vi "Reference - Copy and Paste Buffer.vi"(9 "Cluster2":T1, 10 "Enum":enum16{"Initialize", "Copy", "Paste"}(ring), 11 "DB Refnums":T2) -> (0 "error out":errorcluster)   [LabVIEW 2013]
uses:
  Controls/DB - Refnums.ctl
  Controls/Setup - Part Details - Item Details.ctl
  Controls/Combo Box.ctl
panel:
  out "Array 2":bool[](array[boolean])
  out "Array":bool[](array[boolean])
  out "size(s) 2":i32
  out "size(s)":i32
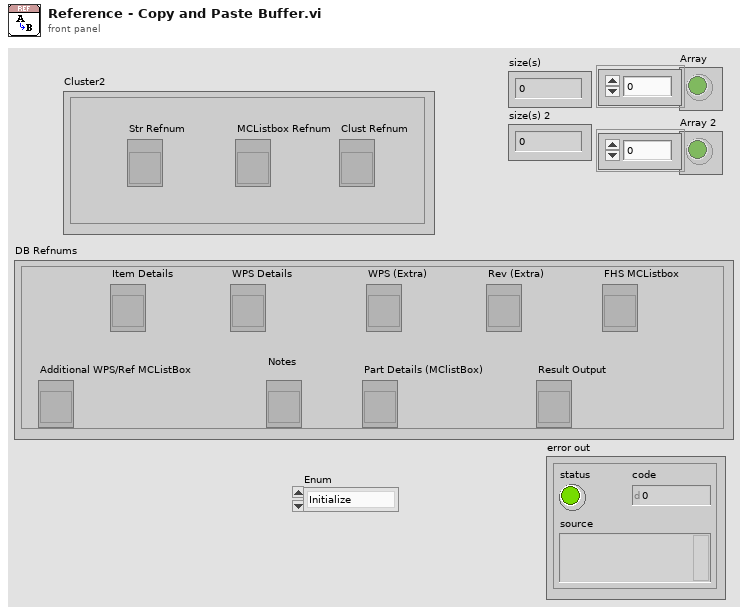
[diagram p1: front panel]
types:
  T1 = cluster{"Str Refnum":refnum<vi>, "MCListbox Refnum":refnum<vi>, "Clust Refnum":refnum<vi>}
  T2 = typedef "DB - Refnums.ctl" = cluster{"Item Details":refnum<vi>, "WPS Details":refnum<vi>, "WPS (Extra)":refnum<vi>, "Rev (Extra) ":refnum<vi>, "FHS MCListbox":refnum<vi>, "Additional WPS/Ref MCListBox":refnum<vi>, "Notes":refnum<vi>, "Part Details (MClistBox)":refnum<vi>, "Result Output":refnum<vi>}
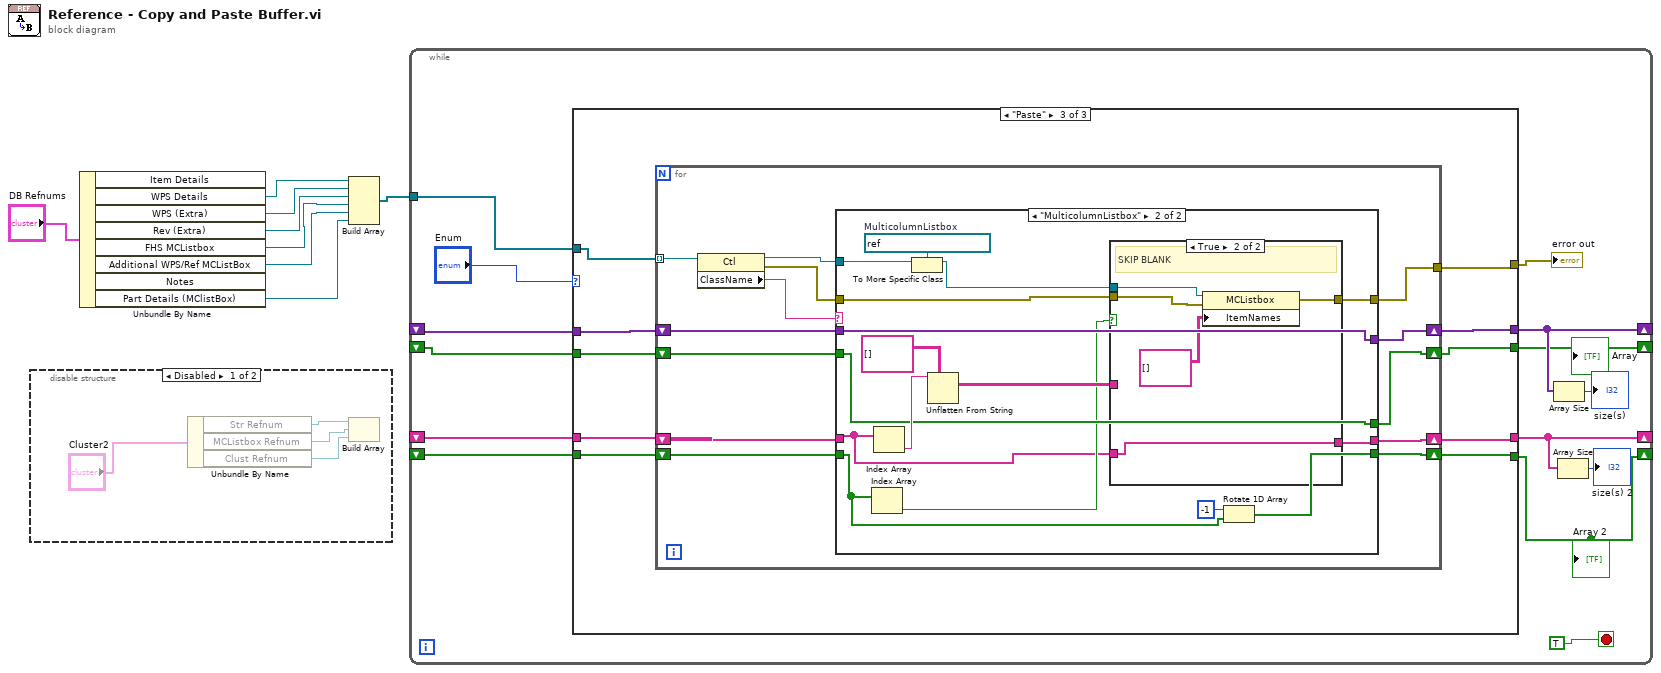
[diagram p0: block diagram]
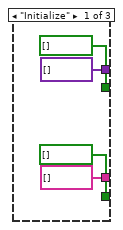
[diagram p3: hidden frame]
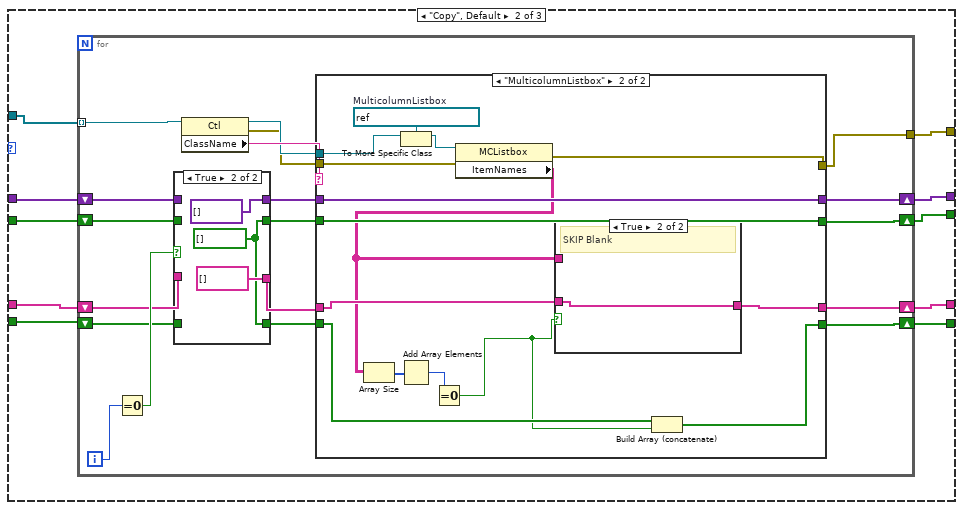
[diagram p4: hidden frame]
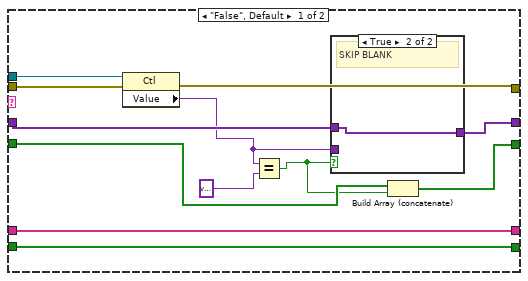
[diagram p6: hidden frame]
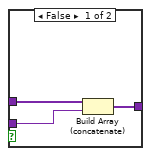
[diagram p7: hidden frame]
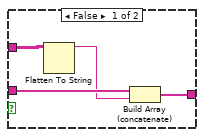
[diagram p8: hidden frame]
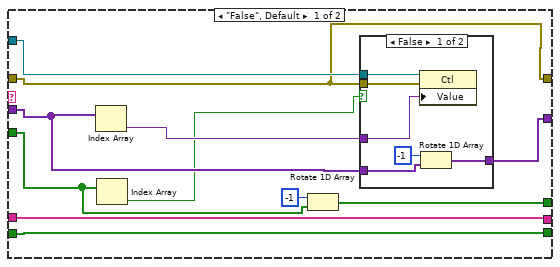
[diagram p9: hidden frame]
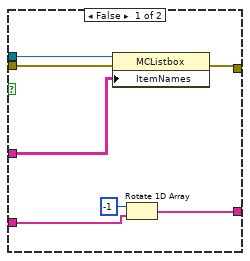
[diagram p11: hidden frame]
diagram:
  n1 = disable-structure shown="Disabled" {
    frame Disabled {
      n2 = Unbundle By Name("Cluster2") -> ("Str Refnum"=w11:refnum<vi>, "MCListbox Refnum"=w10:refnum<vi>, "Clust Refnum"=w9:refnum<vi>)
      n3 = Build Array(w11, w10, w9) -> ()  [unwired: 1 out]
    }
    frame Enabled {
    }
  }
  n4 = Unbundle By Name("DB Refnums") -> ("WPS Details"=w7:refnum<vi>, "WPS (Extra)"=w6:refnum<vi>, "Rev (Extra)"=w5:refnum<vi>, "FHS MCListbox"=w4:refnum<vi>, "Additional WPS/Ref MCListBox"=w3:refnum<vi>, "Part Details (MClistBox)"=w2:refnum<vi>)  [unwired: 2 out]
  n5 = Build Array(w7, w6, w5, w4, w3, w2) -> (w1:refnum<vi>[])
  n6 = while {
    tunnel: w1 -> [w24]
    shift-right: [w20] -> _
    shift-left: _ -> [w23]
    shift-right: [w18] -> _
    shift-left: _ -> [w22]
    shift-right: [w15] -> _
    shift-left: _ -> [w16]
    shift-right: [w13] -> _
    shift-left: _ -> [w14]
    stop <- TRUE stop-if-true
    n7 = case shown="\"Paste\"" "Enum" {
      tunnel: w24 -> [_ w35 w112]
      tunnel: [variant[] [] w40 w109] -> w20
      tunnel: w23 -> [_ w38 w111]
      tunnel: [string[] [] w39 w107] -> w18
      tunnel: w22 -> [_ w37 w108]
      tunnel: [_ w36 w110] -> w21
      tunnel: w16 -> [_ w34 w106]
      tunnel: [bool[] [] w33 w103] -> w15
      tunnel: w14 -> [_ w32 w105]
      tunnel: [bool[] [] w31 w104] -> w13
      frame "Initialize" {
      }
      frame "Copy", Default {
        n8 = for {
          tunnel: w35 -> [w59] mode=indexing
          tunnel: [w53] -> w36
          shift-right: [w54] -> w40
          shift-left: w38 -> [w51]
          shift-right: [w56] -> w39
          shift-left: w37 -> [w49]
          shift-right: [w44] -> w33
          shift-left: w34 -> [w46]
          shift-right: [w41] -> w31
          shift-left: w32 -> [w43]
          i -> [w52]
          n9 = Equal To 0?(x=w52) -> (x = 0?=w50:bool)
          n10 = case shown="True" w50 {
            tunnel: w51 -> [w63 _]
            tunnel: w49 -> [w62 _]
            tunnel: [w63 variant[] []] -> w48
            tunnel: [w62 string[] []] -> w47
            tunnel: w46 -> [w61 _]
            tunnel: [w61 w64] -> w45
            tunnel: w43 -> [w60 _]
            tunnel: [w60 w64] -> w42
            frame False {
            }
            frame True {
              w64 = bool[] []
            }
          }
          n11 = property class="Ctl"(reference=w59) -> (reference out=w57:refnum<vi>, error out=w55:errorcluster, "ClassName"=w58:string)  [unwired: 1 in]
          n12 = case shown="\"MulticolumnListbox\"" w58 {
            tunnel: w57 -> [w78 w97]
            tunnel: [w73 w91] -> w56
            tunnel: w55 -> [w77 w94]
            tunnel: [w76 w93] -> w53
            tunnel: [w74 w90] -> w54
            tunnel: w48 -> [w75 w90]
            tunnel: w47 -> [w73 w92]
            tunnel: w45 -> [w70 w87]
            tunnel: [w68 w87] -> w44
            tunnel: w42 -> [w67 w85]
            tunnel: [w67 w83] -> w41
            frame "False", Default {
              n13 = property class="Ctl"(reference=w78, error in=w77) -> (error out=w76:errorcluster, "Value"=w71:variant)  [unwired: 1 out]
              n14 = Equal?(x=w71, y=variant ("Value")) -> (x = y?=w69:bool)
              n15 = case shown="True" w69 {
                tunnel: w75 -> [w81 w82]
                tunnel: [w80 w82] -> w74
                tunnel: w71 -> [w79 _]
                frame False {
                  n16 = Build Array (concatenate)(w81, w79) -> (w80:variant[])
                }
                frame True {
                  # "SKIP BLANK"
                }
              }
              n17 = Build Array (concatenate)(w70, w69) -> (w68:bool[])
            }
            frame "MulticolumnListbox" {
              w95 = refnum<vi> refnum  # MulticolumnListbox
              n18 = To More Specific Class(target class=w95, reference=w97) -> (specific class reference=w96:refnum<vi>)  [unwired: 1 in, 1 out]
              n19 = property class="MCListbox"(reference=w96, error in=w94) -> (error out=w93:errorcluster, "ItemNames"=w86:string[][])  [unwired: 1 out]
              n20 = Array Size(array=w86) -> (size(s)=w89:i32[])
              n21 = Add Array Elements(numeric array=w89) -> (sum=w88:i32)
              n22 = Equal To 0?(x=w88) -> (x = 0?=w84:bool)
              n23 = case shown="True" w84 {
                tunnel: w92 -> [w101 w102]
                tunnel: [w99 w102] -> w91
                tunnel: w86 -> [w98 _]
                frame False {
                  n24 = Flatten To String(anything=w98) -> (data string=w100:string)  [unwired: 3 in, 2 out]
                  n25 = Build Array (concatenate)(w101, w100) -> (w99:string[])
                }
                frame True {
                  # "SKIP Blank"
                }
              }
              n26 = Build Array (concatenate)(w85, w84) -> (w83:bool[])
            }
          }
        }
      }
      frame "Paste" {
        n27 = for {
          tunnel: w112 -> [w125] mode=indexing
          tunnel: [w121] -> w110
          shift-right: [w119] -> w109
          shift-left: w111 -> [w120]
          shift-right: [w117] -> w107
          shift-left: w108 -> [w118]
          shift-right: [w115] -> w103
          shift-left: w106 -> [w116]
          shift-right: [w113] -> w104
          shift-left: w105 -> [w114]
          n28 = property class="Ctl"(reference=w125) -> (reference out=w123:refnum<vi>, error out=w122:errorcluster, "ClassName"=w124:string)  [unwired: 1 in]
          n29 = case shown="\"MulticolumnListbox\"" w124 {
            tunnel: w118 -> [w135 w148]
            tunnel: w123 -> [w136 w157]
            tunnel: w122 -> [w133 w156]
            tunnel: [w133 w155] -> w121
            tunnel: w120 -> [w131 w153]
            tunnel: [w130 w153] -> w119
            tunnel: [w135 w147] -> w117
            tunnel: w116 -> [w128 w151]
            tunnel: [w127 w151] -> w115
            tunnel: w114 -> [w126 w145]
            tunnel: [w126 w144] -> w113
            frame "False", Default {
              n30 = Index Array(array=w131) -> (element=w134:variant)  [unwired: 1 in]
              n31 = Index Array(array=w128) -> (element=w129:bool)  [unwired: 1 in]
              n32 = Rotate 1D Array(1:w128, 2:-1 ("n")) -> (0:w127:bool[])
              n33 = case shown="False" w129 {
                tunnel: w136 -> [w142 _]
                tunnel: w134 -> [w141 _]
                tunnel: w133 -> [w140 _]
                tunnel: w131 -> [w138 w143]
                tunnel: [w137 w143] -> w130
                frame False {
                  n34 = property class="Ctl"(reference=w142, error in=w140, "Value"=w141) -> ()  [unwired: 2 out]
                  n35 = Rotate 1D Array(1:w138, 2:-1 ("n")) -> (0:w137:variant[])
                }
                frame True {
                  # "SKIP"
                }
              }
            }
            frame "MulticolumnListbox" {
              w158 = refnum<vi> refnum  # MulticolumnListbox
              n36 = Index Array(array=w145) -> (element=w149:bool)  [unwired: 1 in]
              n37 = Index Array(array=w148) -> (element=w152:string)  [unwired: 1 in]
              n38 = To More Specific Class(target class=w158, reference=w157) -> (specific class reference=w159:refnum<vi>)  [unwired: 1 in, 1 out]
              n39 = Unflatten From String(type=string[][] [], binary string=w152) -> (value=w150:string[][])  [unwired: 3 in, 2 out]
              n40 = case shown="True" w149 {
                tunnel: w159 -> [w166 w167]
                tunnel: w156 -> [w165 w170]
                tunnel: [w164 w169] -> w155
                tunnel: w150 -> [w163 _]
                tunnel: w148 -> [w161 w171]
                tunnel: [w160 w171] -> w147
                frame False {
                  n41 = property class="MCListbox"(reference=w166, error in=w165, "ItemNames"=w163) -> (error out=w164:errorcluster)  [unwired: 1 out]
                  n42 = Rotate 1D Array(1:w161, 2:-1 ("n")) -> (0:w160:string[])
                }
                frame True {
                  # "SKIP BLANK"
                  n43 = property class="MCListbox"(reference=w167, error in=w170, "ItemNames"=string[][] []) -> (error out=w169:errorcluster)  [unwired: 1 out]
                }
              }
              n44 = Rotate 1D Array(1:w145, 2:-1 ("n")) -> (0:w144:bool[])
            }
          }
        }
      }
    }
    "error out" <- w21
    "Array" <- w15
    "Array 2" <- w13
    n45 = Array Size(array=w20) -> (size(s)=→"size(s)":i32)
    n46 = Array Size(array=w18) -> (size(s)=→"size(s) 2":i32)
  }
